vi "Create Write Channel.vi"(7 "Name":string, 8 "error in (no error)":errorcluster, 9 "Cluster":T1 {"Data Type" format="%.0x"}, 10 "Bitfile Name":string, 11 "Item Ref in":T3 format="%.0x") -> (0 "error out":errorcluster)   [LabVIEW 2018, in "FPGA Addon System Explorer.lvlib"]
uses:
  FPGA Addon System Explorer.lvlib
  <vilib>/NI Veristand/Custom Device API/Custom Device Item Ref.ctl
  Addon Shared/Types/Register Information.ctl
  Addon Shared/Types/Data Type.ctl
  <vilib>/NI Veristand/Custom Device API/Custom Device Channel.ctl
  <vilib>/NI Veristand/Custom Device API/Custom Device Channel Type.ctl
  Addon Shared/Types/FG Action.ctl
  niveristand-fpga-addon-speciality-io/Source/Types/PWM.Measure.Analog.Settings.ctl
  niveristand-fpga-addon-speciality-io/Source/Types/PWM.Generate.Digital.Convert.Settings.ctl
  niveristand-fpga-addon-speciality-io/Source/Types/PWM.Generate.Digital.Settings.ctl
  niveristand-fpga-addon-speciality-io/Source/Types/WSS.Generate.Digital.Convert.Settings.ctl
  niveristand-fpga-addon-speciality-io/Source/Types/WSS.Generate.Digital.Settings.ctl
  niveristand-fpga-addon-speciality-io/Source/Types/WSS.Sensor.Type.ctl
  niveristand-fpga-addon-speciality-io/Source/Types/Static.Generate.Digital.Settings.ctl
  niveristand-fpga-addon-speciality-io/Source/Types/Static.Measure.Digital.Settings.ctl
  niveristand-fpga-addon-speciality-io/Source/Types/Sine.Generate.Convert.Settings.ctl
  niveristand-fpga-addon-speciality-io/Source/Types/Sine.Generate.Settings.ctl
  niveristand-fpga-addon-speciality-io/Source/Types/PWM.Measure.Digital.Settings.ctl
  niveristand-fpga-addon-speciality-io/Source/Types/QuadratureEncoder.Measure.Digital.Settings.ctl
  niveristand-fpga-addon-speciality-io/Source/Types/QuadratureEncoder.Measure.Digital.Settings.Direction.ctl
  Addon Shared/SubVIs/Constants.vi
  <vilib>/NI/NI VeriStand Advanced SysDef API/SysDef API/SysDef.Property.Get.vi
  <vilib>/NI/NI VeriStand Advanced SysDef API/_SubVIs/SysDef.Property.Get.Variant.vi
  <vilib>/NI/NI VeriStand Advanced SysDef API/SysDef API/SysDef.Property.Set.vi
  <vilib>/NI/NI VeriStand Advanced SysDef API/_SubVIs/SysDef.Property.Set.Variant.vi
  <vilib>/NI Veristand/Custom Device API/Custom Device API.lvlib
  Addon Shared/FPGA Addon Shared.lvlib
  niveristand-fpga-addon-speciality-io/Source/Speciality FPGA IO.lvlib
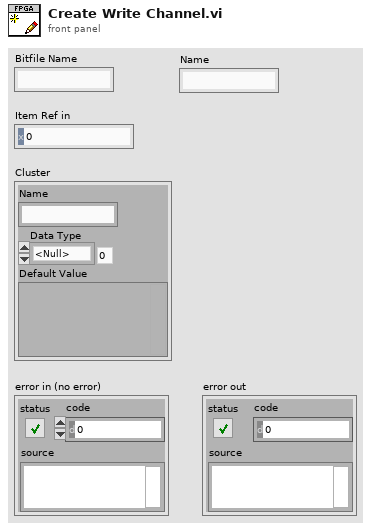
[diagram p1: front panel]
types:
  T1 = typedef "FPGA Addon Shared.lvlib/Register Information.ctl" = cluster{"Name":string, "Data Type":T2, "Default Value":variant}
  T2 = typedef "FPGA Addon Shared.lvlib/Data Type.ctl" = enum8{"<Null>", "I8", "I16", "I32", "I64", "U8", "U16", "U32", "U64", "SGL", "Boolean", "Analog PWM In Settings", "Analog PWM In", "Digital PWM In Settings", "Digital PWM In", "Digital PWM Out", "Sine Out", "FXP+/-24.5", "FXP+/-16.5", "FXP+/-32.8", "FXP+/-64.32", "FXP+/-16.7", "FXP+/-20.5", "FXP+/-27.5", "FXP+/-32.16", "FXP+16.3", "FXP+18.3", "Digital Static In", "Digital Static Out", "Digital Static In Settings", "Digital WSS Out", "Quad Encoder Settings", "Quad Encoder In", "Group"}
  T3 = typedef "Custom Device API.lvlib/Custom Device Item Ref.ctl" = u64
  T4 = typedef "Custom Device API.lvlib/Custom Device Channel.ctl" = cluster{"Type":T5, "Units":string, "Default Value":dbl, "Faultable":bool, "Scalable":bool}
  T5 = typedef "Custom Device API.lvlib/Custom Device Channel Type.ctl" = enum16{"Input", "Output"}
  T6 = typedef "FPGA Addon Shared.lvlib/FG Action.ctl" = enum8{"GET", "SET"}
  T7 = typedef "Speciality FPGA IO.lvlib/PWM.Measure.Analog.Settings.ctl" = cluster{"ACTIVE EDGE":bool, "TIMEOUT":u32, "THRESHOLD":fxp<+/-,32,8>}
  T8 = typedef "Speciality FPGA IO.lvlib/PWM.Generate.Digital.Convert.Settings.ctl" = cluster{"ACTIVE EDGE":bool, "FREQ":sgl, "DC":sgl}
  T9 = typedef "Speciality FPGA IO.lvlib/PWM.Generate.Digital.Settings.ctl" = cluster{"ACTIVE EDGE":bool, "ACTIVE TICKS":u32, "INACTIVE TICKS":u32}
  T10 = typedef "Speciality FPGA IO.lvlib/WSS.Generate.Digital.Convert.Settings.ctl" = cluster{"SPEED":u32, "DATA":u8, "PPR":u32, "WD":u32, "TYPE":u8}
  T11 = typedef "Speciality FPGA IO.lvlib/WSS.Generate.Digital.Settings.ctl" = cluster{"ACTIVE EDGE":bool, "ACTIVE TICKS":u32, "INACTIVE TICKS":u32, "DATA":u8, "SENSOR TYPE":u8}
  T12 = typedef "Speciality FPGA IO.lvlib/WSS.Sensor.Type.ctl" = enum16{"Unidirectional", "Bosch Bidirectional", "Continental Bidirectional"}
  T13 = typedef "Speciality FPGA IO.lvlib/Sine.Generate.Convert.Settings.ctl" = cluster{"AMP":sgl, "OFFSET":sgl, "FREQ":sgl}
  T14 = typedef "Speciality FPGA IO.lvlib/Sine.Generate.Settings.ctl" = cluster{"AMP":fxp<+/-,32,8>, "OFFSET":fxp<+/-,32,8>, "PERIODS/TICKS":fxp<+,32,0>}
  T15 = typedef "Speciality FPGA IO.lvlib/QuadratureEncoder.Measure.Digital.Settings.Direction.ctl" = enum16{"Increment A Leads B", "Increment B Leads A"}
  T16 = typedef "Speciality FPGA IO.lvlib/Static.Generate.Digital.Settings.ctl" = cluster{"ACTIVE EDGE":bool, "OUTPUT":bool}
  T17 = typedef "Speciality FPGA IO.lvlib/Static.Measure.Digital.Settings.ctl" = cluster{"ACTIVE EDGE":bool}
  T18 = typedef "Speciality FPGA IO.lvlib/PWM.Measure.Digital.Settings.ctl" = cluster{"ACTIVE EDGE":bool, "TIMEOUT":u32}
  T19 = typedef "Speciality FPGA IO.lvlib/QuadratureEncoder.Measure.Digital.Settings.ctl" = cluster{"DIRECTION":u8, "RESET VALUE":i32, "A RESET STATE":bool, "B RESET STATE":bool, "Z RESET STATE":bool}
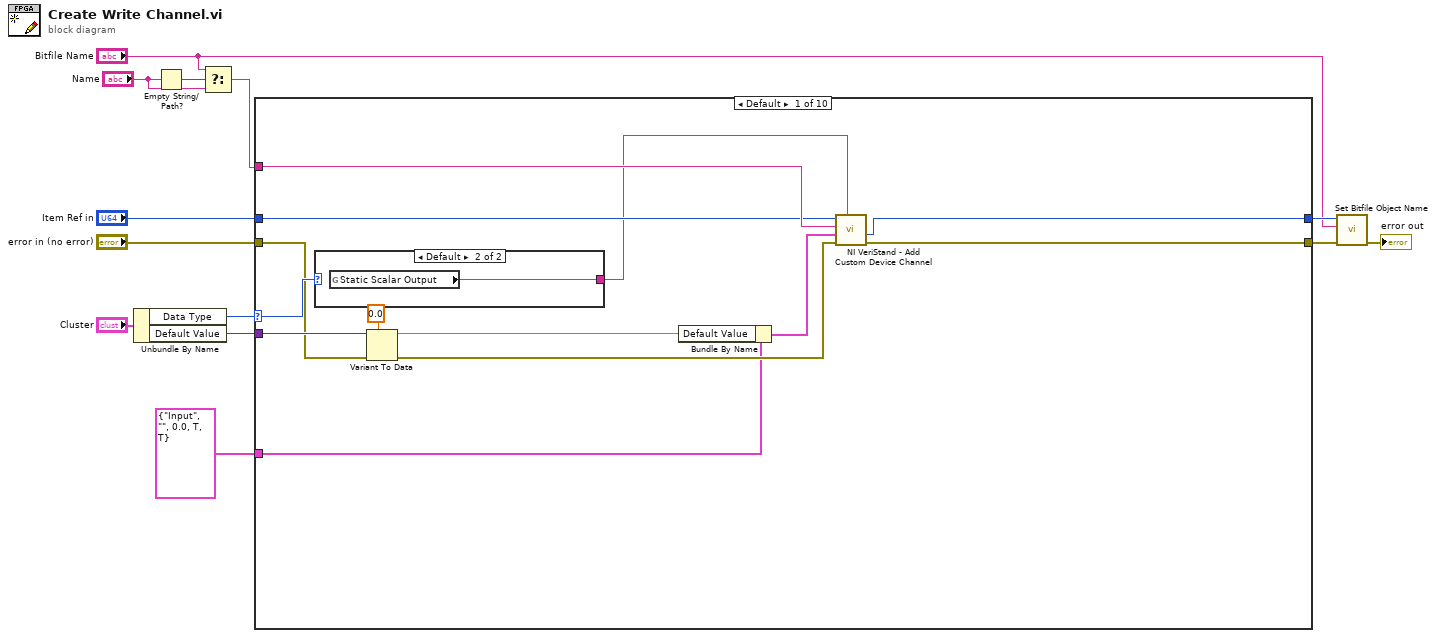
[diagram p0: block diagram]
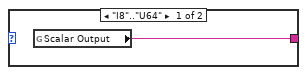
[diagram p2: hidden frame]
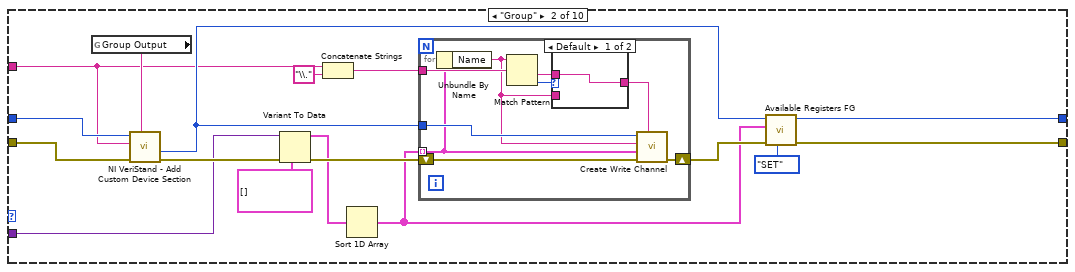
[diagram p3: hidden frame]
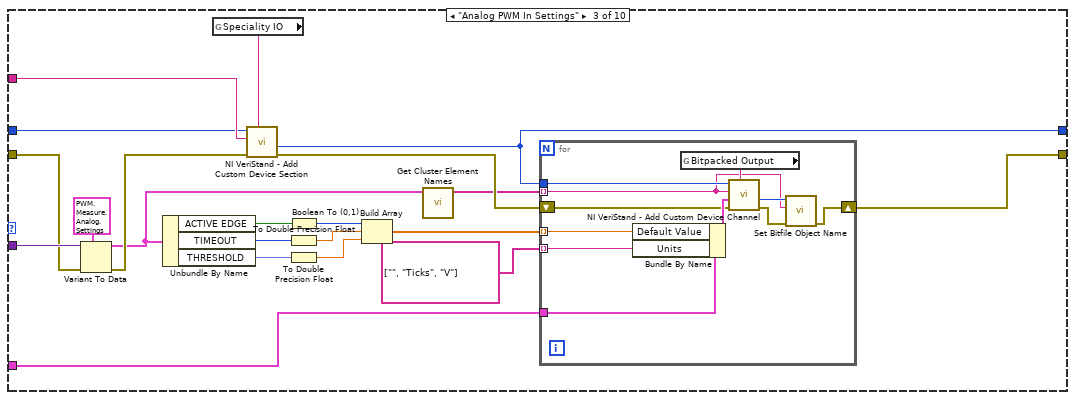
[diagram p5: hidden frame]
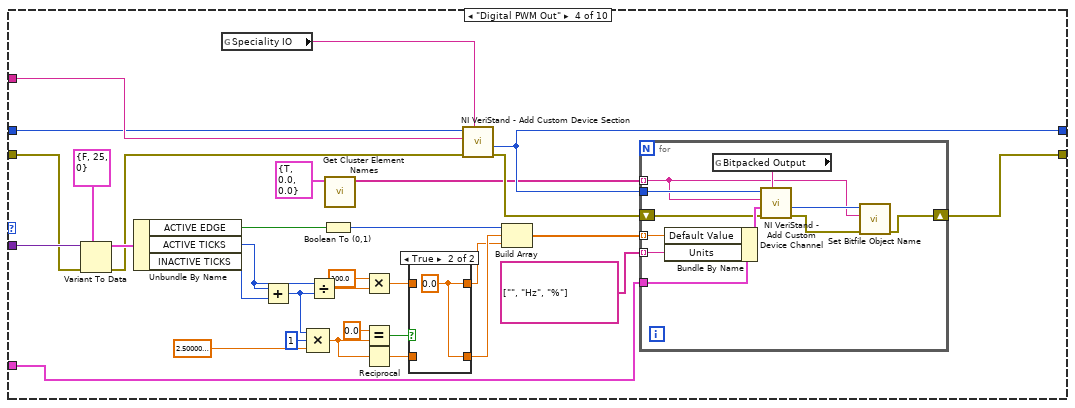
[diagram p6: hidden frame]
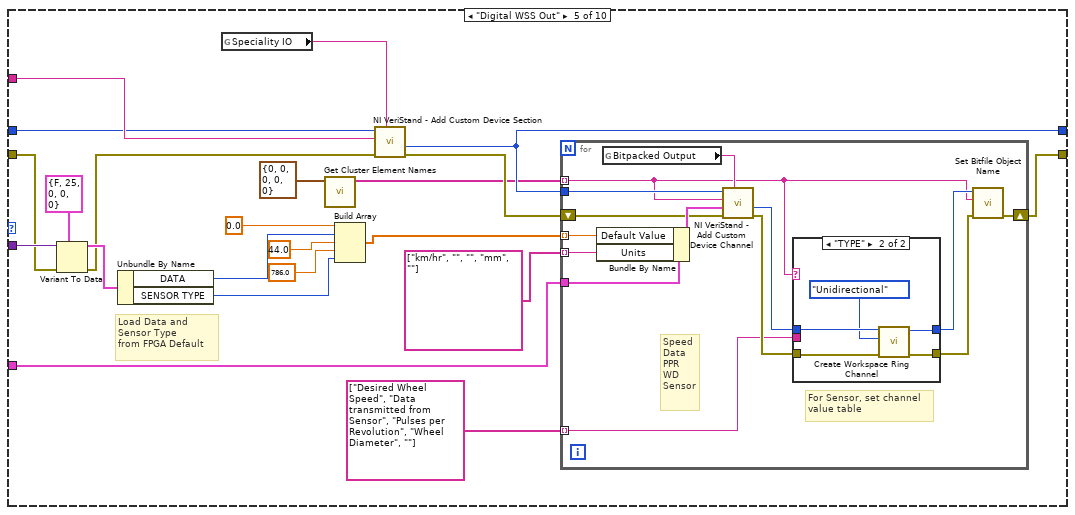
[diagram p8: hidden frame]
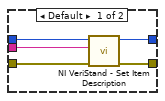
[diagram p9: hidden frame]
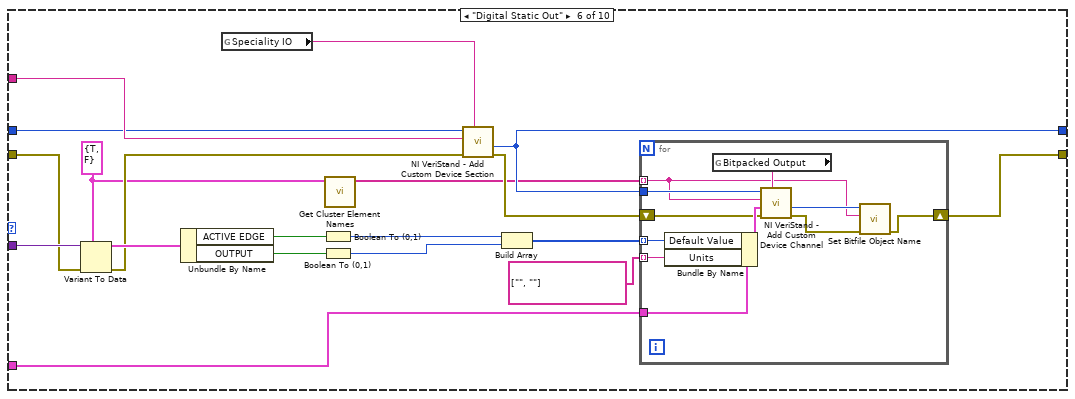
[diagram p10: hidden frame]
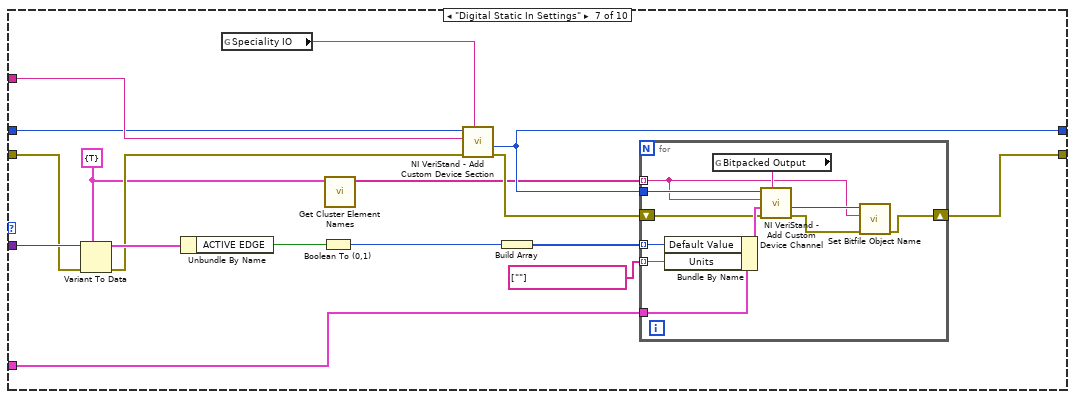
[diagram p11: hidden frame]
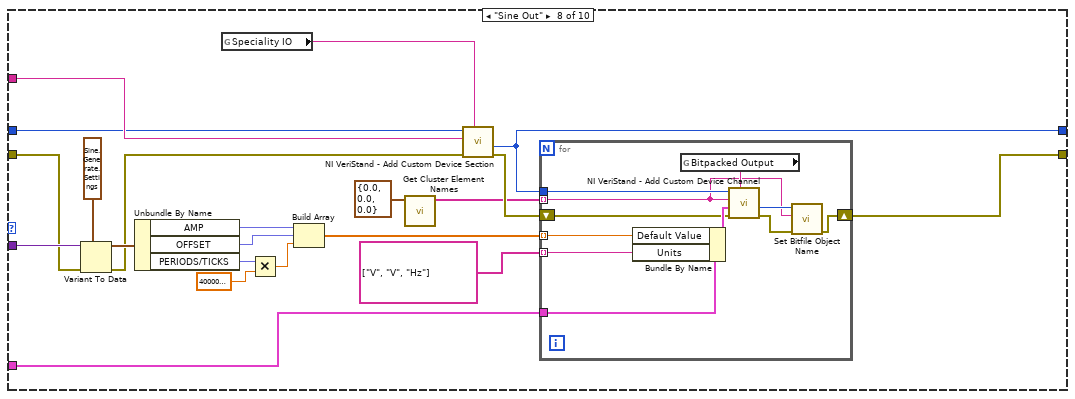
[diagram p12: hidden frame]
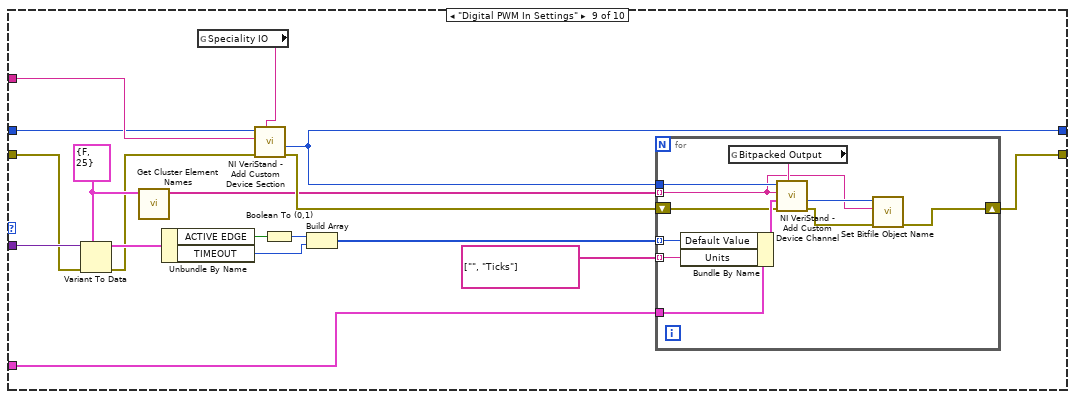
[diagram p13: hidden frame]
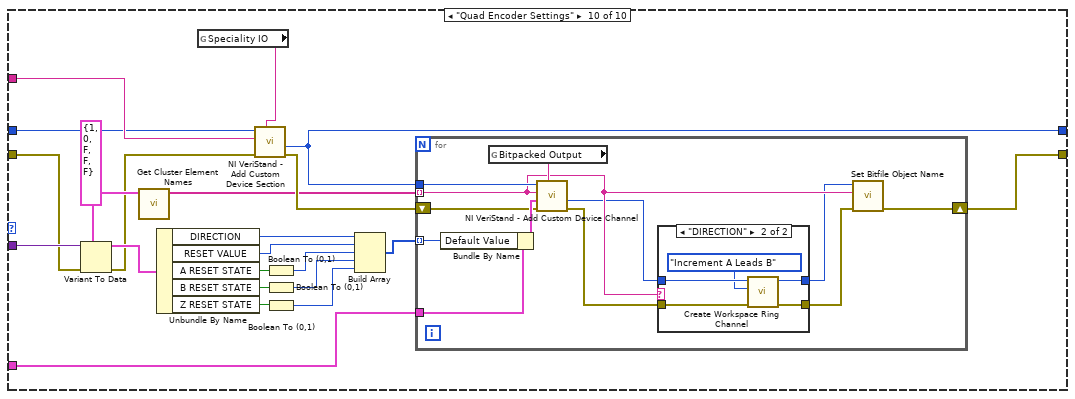
[diagram p14: hidden frame]
diagram:
  n1 = Unbundle By Name("Cluster") -> ("Data Type"=w9:T2, "Default Value"=w8:variant)
  n2 = Empty String/Path?(string/path="Name") -> (empty?=w4:bool)
  n3 = Select(t="Bitfile Name", s=w4, f="Name") -> (s? t:f=w1:string)
  n4 = case shown="Default" w9 {
    selector: w9 -> [w20 _ _ _ _ _ _ _ _ _]
    tunnel: [w26 w34 w71 w114 w150 w193 w221 w253 w282 w315] -> w12
    tunnel: w1 -> [w25 w30 w77 w120 w156 w199 w227 w259 w288 w321]
    tunnel: [w24 w36 w70 w116 w152 w195 w223 w255 w284 w317] -> w11
    tunnel: "Item Ref in" -> [w23 w40 w76 w119 w155 w198 w226 w258 w287 w320]
    tunnel: "error in (no error)" -> [w16 w41 w74 w117 w153 w196 w224 w256 w285 w318]
    tunnel: w8 -> [w19 w39 w75 w118 w154 w197 w225 w257 w286 w319]
    tunnel: T4 {"Type"=enum."Input", "Units"="", "Default Value"=0.0, "Faultable"=TRUE, "Scalable"=TRUE} ("Channel") -> [w14 _ w57 w89 w141 w181 w211 w239 w271 w307]
    frame Default {
      n5 = case shown="Default" w20 {
        tunnel: [w27 w28] -> w22
        frame "I8".."U64" {
          n6 = global read "Constants.vi" "Scalar Output"() -> (w27:string)
        }
        frame Default {
          n7 = global read "Constants.vi" "Static Scalar Output"() -> (w28:string)
        }
      }
      n8 = Variant To Data(error in=w16, type=0.0 ("Default Value"), Variant=w19) -> (data=w17:dbl, error out=w15:errorcluster)
      n9 = Bundle By Name(cluster=w14, "Default Value"=w17) -> (w21:T4)
      n10 = call <vilib>:"NI VeriStand - Add Custom Device Channel.vi"("GUID (Default Channel)"=w22, "error in (no error)"=w15, "Channel"=w21, "Channel Name"=w25, "Parent Ref in"=w23) -> ("error out"=w26:errorcluster, "Channel Ref"=w24:T3)  [unwired: 3 in, 2 out]
    }
    frame "Group" {
      n11 = global read "Constants.vi" "Group Output"() -> (w43:string)
      n12 = call <vilib>:"NI VeriStand - Add Custom Device Section.vi"("GUID (Default Section)"=w43, "error in (no error)"=w41, "Section Name"=w30, "Parent Ref in"=w40) -> ("error out"=w42:errorcluster, "Section Ptr"=w37:T3)  [unwired: 4 in, 2 out]
      n13 = Variant To Data(error in=w42, type=T1[] [], Variant=w39) -> (data=w33:T1[], error out=w44:errorcluster)
      n14 = Concatenate Strings(w30, "\\.") -> (w29:string)
      n15 = Sort 1D Array(array=w33) -> (sorted array=w32:T1[])
      n16 = for {
        tunnel: w32 -> [w48] mode=indexing
        shift-right: [w52] -> w35
        shift-left: w44 -> [w54]
        tunnel: w37 -> [w53]
        tunnel: w29 -> [w49]
        n17 = Unbundle By Name(w48) -> ("Name"=w47:string)
        n18 = Match Pattern(string=w47, regular expression=w49) -> (after substring=w50:string, offset past match=w51:i32)  [unwired: 1 in, 2 out]
        n19 = case shown="Default" w51 {
          tunnel: [w55 w56] -> w46
          tunnel: w50 -> [w55 _]
          tunnel: w47 -> [_ w56]
          frame Default {
          }
          frame -1 {
          }
        }
        n20 = call "Create Write Channel.vi"("Name"=w46, "error in (no error)"=w54, "Cluster"=w48, "Bitfile Name"=w47, "Item Ref in"=w53) -> ("error out"=w52:errorcluster)  [unwired: 6 in]
      }
      n21 = call "Available Registers FG.vi"("Action"=FG_Action."SET", "error in (no error)"=w35, "Available Registers"=w32, "Item Ref"=w37) -> ("error out"=w34:errorcluster, "Item Ref out"=w36:T3)  [unwired: 5 in, 1 out]
    }
    frame "Analog PWM In Settings" {
      n22 = Variant To Data(error in=w74, type=T7 {"ACTIVE EDGE"=FALSE, "TIMEOUT"=1000000000, "THRESHOLD"=25.0} ("Channel.Settings"), Variant=w75) -> (data=w59:T7, error out=w60:errorcluster)
      n23 = Unbundle By Name(w59) -> ("ACTIVE EDGE"=w65:bool, "TIMEOUT"=w69:u32, "THRESHOLD"=w64:fxp<+/-,32,8>)
      n24 = global read "Constants.vi" "Speciality IO"() -> (w61:string)
      n25 = call <vilib>:"NI VeriStand - Add Custom Device Section.vi"("GUID (Default Section)"=w61, "error in (no error)"=w60, "Section Name"=w77, "Parent Ref in"=w76) -> ("error out"=w72:errorcluster, "Section Ptr"=w70:T3)  [unwired: 4 in, 2 out]
      n26 = Boolean To (0,1)(Boolean=w65) -> (0, 1=w63:i16)
      n27 = To Double Precision Float(number=w69) -> (double precision float=w67:dbl)
      n28 = To Double Precision Float(number=w64) -> (double precision float=w62:dbl)
      n29 = Build Array(w63, w67, w62) -> (w68:dbl[])
      n30 = call "Get Cluster Element Names.vi"("Cluster"=w59) -> ("Channels"=w58:string[])  [unwired: 10 in]
      n31 = for {
        tunnel: w70 -> [w87]
        shift-right: [w80] -> w71
        shift-left: w72 -> [w86]
        tunnel: w68 -> [w84] mode=indexing
        tunnel: string[] ["", "Ticks", "V"] -> [w83] mode=indexing
        tunnel: w58 -> [w79] mode=indexing
        tunnel: w57 -> [w78]
        n32 = Bundle By Name(cluster=w78, "Default Value"=w84, "Units"=w83) -> (w88:T4)
        n33 = global read "Constants.vi" "Bitpacked Output"() -> (w85:string)
        n34 = call <vilib>:"NI VeriStand - Add Custom Device Channel.vi"("GUID (Default Channel)"=w85, "error in (no error)"=w86, "Channel"=w88, "Channel Name"=w79, "Parent Ref in"=w87) -> ("error out"=w81:errorcluster, "Channel Ref"=w82:T3)  [unwired: 3 in, 2 out]
        n35 = call "Set Bitfile Object Name.vi"("error in (no error)"=w81, "Name"=w79, "Channel Ref"=w82) -> ("error out"=w80:errorcluster)  [unwired: 8 in]
      }
    }
    frame "Digital PWM Out" {
      n36 = Variant To Data(error in=w117, type=T9 {"ACTIVE EDGE"=FALSE, "ACTIVE TICKS"=25, "INACTIVE TICKS"=0} ("Channel.Settings"), Variant=w118) -> (data=w113:T9, error out=w106:errorcluster)
      n37 = Unbundle By Name(w113) -> ("ACTIVE EDGE"=w112:bool, "ACTIVE TICKS"=w97:u32, "INACTIVE TICKS"=w96:u32)
      n38 = global read "Constants.vi" "Speciality IO"() -> (w109:string)
      n39 = Add(x=w97, y=w96) -> (x+y=w103:u32)
      n40 = Compound Arithmetic op=MULTIPLY(w103, u32 1 ("value"), 2.5000000292152436e-08 ("y")) -> (w104:dbl)
      n41 = Divide(x=w97, y=w103) -> (x/y=w99:dbl)
      n42 = Boolean To (0,1)(Boolean=w112) -> (0, 1=w111:i16)
      n43 = call "Get Cluster Element Names.vi"("Cluster"=T8 {"ACTIVE EDGE"=TRUE, "FREQ"=0.0, "DC"=0.0} ("Settings")) -> ("Channels"=w107:string[])  [unwired: 10 in]
      n44 = Multiply(x=100.0, y=w99) -> (x*y=w91:dbl)
      n45 = Equal?(x=0.0, y=w104) -> (x = y?=w95:bool)
      n46 = Reciprocal(x=w104) -> (1/x=w93:dbl)
      n47 = case shown="True" w95 {
        tunnel: [w122 w123] -> w94
        tunnel: w93 -> [w122 _]
        tunnel: [w121 w123] -> w92
        tunnel: w91 -> [w121 _]
        frame False {
        }
        frame True {
          w123 = 0.0
        }
      }
      n48 = call <vilib>:"NI VeriStand - Add Custom Device Section.vi"("GUID (Default Section)"=w109, "error in (no error)"=w106, "Section Name"=w120, "Parent Ref in"=w119) -> ("error out"=w115:errorcluster, "Section Ptr"=w116:T3)  [unwired: 4 in, 2 out]
      n49 = Build Array(w111, w94, w92) -> (w110:dbl[])
      n50 = for {
        tunnel: w116 -> [w133]
        shift-right: [w126] -> w114
        shift-left: w115 -> [w132]
        tunnel: w110 -> [w130] mode=indexing
        tunnel: w107 -> [w125] mode=indexing
        tunnel: string[] ["", "Hz", "%"] -> [w129] mode=indexing
        tunnel: w89 -> [w124]
        n51 = Bundle By Name(cluster=w124, "Default Value"=w130, "Units"=w129) -> (w134:T4)
        n52 = global read "Constants.vi" "Bitpacked Output"() -> (w131:string)
        n53 = call <vilib>:"NI VeriStand - Add Custom Device Channel.vi"("GUID (Default Channel)"=w131, "error in (no error)"=w132, "Channel"=w134, "Channel Name"=w125, "Parent Ref in"=w133) -> ("error out"=w127:errorcluster, "Channel Ref"=w128:T3)  [unwired: 3 in, 2 out]
        n54 = call "Set Bitfile Object Name.vi"("error in (no error)"=w127, "Name"=w125, "Channel Ref"=w128) -> ("error out"=w126:errorcluster)  [unwired: 8 in]
      }
    }
    frame "Digital WSS Out" {
      # "Load Data and\nSensor Type\nfrom FPGA Default"
      n55 = Variant To Data(error in=w153, type=T11 {"ACTIVE EDGE"=FALSE, "ACTIVE TICKS"=25, "INACTIVE TICKS"=0, "DATA"=0, "SENSOR TYPE"=0} ("Channel.Settings"), Variant=w154) -> (data=w149:T11, error out=w144:errorcluster)
      n56 = Unbundle By Name(w149) -> ("DATA"=w135:u8, "SENSOR TYPE"=w136:u8)
      n57 = global read "Constants.vi" "Speciality IO"() -> (w147:string)
      n58 = call "Get Cluster Element Names.vi"("Cluster"=T10 {"SPEED"=0, "DATA"=0, "PPR"=0, "WD"=0, "TYPE"=0} ("Wheel Speed Sensor Settings")) -> ("Channels"=w145:string[])  [unwired: 10 in]
      n59 = Build Array(0.0 ("element"), w135, 44.0 ("element"), 786.0 ("element"), w136) -> (w148:dbl[])
      n60 = call <vilib>:"NI VeriStand - Add Custom Device Section.vi"("GUID (Default Section)"=w147, "error in (no error)"=w144, "Section Name"=w156, "Parent Ref in"=w155) -> ("error out"=w151:errorcluster, "Section Ptr"=w152:T3)  [unwired: 4 in, 2 out]
      n61 = for {
        tunnel: w152 -> [w169]
        shift-right: [w164] -> w150
        shift-left: w151 -> [w168]
        tunnel: w148 -> [w166] mode=indexing
        tunnel: w145 -> [w157] mode=indexing
        tunnel: string[] ["km/hr", "", "", "mm", ""] -> [w165] mode=indexing
        tunnel: w141 -> [w163]
        tunnel: string[] ["Desired Wheel Speed", "Data transmitted from Sensor", "Pulses per Revolution", "Wheel Diameter", ""] -> [w158] mode=indexing
        # "For Sensor, set channel \nvalue table"
        # "Speed\nData\nPPR\nWD\nSensor"
        n62 = Bundle By Name(cluster=w163, "Default Value"=w166, "Units"=w165) -> (w170:T4)
        n63 = global read "Constants.vi" "Bitpacked Output"() -> (w167:string)
        n64 = call <vilib>:"NI VeriStand - Add Custom Device Channel.vi"("GUID (Default Channel)"=w167, "error in (no error)"=w168, "Channel"=w170, "Channel Name"=w157, "Parent Ref in"=w169) -> ("error out"=w162:errorcluster, "Channel Ref"=w160:T3)  [unwired: 3 in, 2 out]
        n65 = case shown="\"TYPE\"" w157 {
          tunnel: w162 -> [w175 w179]
          tunnel: [w174 w178] -> w161
          tunnel: w160 -> [w173 w180]
          tunnel: [w172 w177] -> w159
          tunnel: w158 -> [w171 _]
          frame Default {
            n66 = call <vilib>:"NI VeriStand - Set Item Description.vi"("error in (no error)"=w175, "Description"=w171, "Item Ref in"=w173) -> ("error out"=w174:errorcluster, "Item Ref out"=w172:T3)  [unwired: 6 in, 1 out]
          }
          frame "TYPE" {
            n67 = call "Create Workspace Ring Channel.vi"("error in (no error)"=w179, "Enum"=WSS.Sensor.Type."Unidirectional" ("Sensor Type"), "Channel Ref in"=w180) -> ("error out"=w178:errorcluster, "Channel Ref out"=w177:T3)  [unwired: 7 in]
          }
        }
        n68 = call "Set Bitfile Object Name.vi"("error in (no error)"=w161, "Name"=w157, "Channel Ref"=w159) -> ("error out"=w164:errorcluster)  [unwired: 8 in]
      }
    }
    frame "Digital Static Out" {
      w184 = T16 {"ACTIVE EDGE"=TRUE, "OUTPUT"=FALSE} ("Settings")
      n69 = Variant To Data(error in=w196, type=w184, Variant=w197) -> (data=w192:T16, error out=w186:errorcluster)
      n70 = Unbundle By Name(w192) -> ("ACTIVE EDGE"=w191:bool, "OUTPUT"=w183:bool)
      n71 = global read "Constants.vi" "Speciality IO"() -> (w188:string)
      n72 = Boolean To (0,1)(Boolean=w191) -> (0, 1=w190:i16)
      n73 = Boolean To (0,1)(Boolean=w183) -> (0, 1=w182:i16)
      n74 = call "Get Cluster Element Names.vi"("Cluster"=w184) -> ("Channels"=w187:string[])  [unwired: 10 in]
      n75 = call <vilib>:"NI VeriStand - Add Custom Device Section.vi"("GUID (Default Section)"=w188, "error in (no error)"=w186, "Section Name"=w199, "Parent Ref in"=w198) -> ("error out"=w194:errorcluster, "Section Ptr"=w195:T3)  [unwired: 4 in, 2 out]
      n76 = Build Array(w190, w182) -> (w189:i16[])
      n77 = for {
        tunnel: w195 -> [w209]
        shift-right: [w202] -> w193
        shift-left: w194 -> [w208]
        tunnel: w189 -> [w206] mode=indexing
        tunnel: w187 -> [w201] mode=indexing
        tunnel: string[] ["", ""] -> [w205] mode=indexing
        tunnel: w181 -> [w200]
        n78 = Bundle By Name(cluster=w200, "Default Value"=w206, "Units"=w205) -> (w210:T4)
        n79 = global read "Constants.vi" "Bitpacked Output"() -> (w207:string)
        n80 = call <vilib>:"NI VeriStand - Add Custom Device Channel.vi"("GUID (Default Channel)"=w207, "error in (no error)"=w208, "Channel"=w210, "Channel Name"=w201, "Parent Ref in"=w209) -> ("error out"=w203:errorcluster, "Channel Ref"=w204:T3)  [unwired: 3 in, 2 out]
        n81 = call "Set Bitfile Object Name.vi"("error in (no error)"=w203, "Name"=w201, "Channel Ref"=w204) -> ("error out"=w202:errorcluster)  [unwired: 8 in]
      }
    }
    frame "Digital Static In Settings" {
      w212 = T17 {"ACTIVE EDGE"=TRUE} ("Settings")
      n82 = Variant To Data(error in=w224, type=w212, Variant=w225) -> (data=w220:T17, error out=w214:errorcluster)
      n83 = Unbundle By Name(w220) -> ("ACTIVE EDGE"=w219:bool)
      n84 = global read "Constants.vi" "Speciality IO"() -> (w216:string)
      n85 = Boolean To (0,1)(Boolean=w219) -> (0, 1=w218:i16)
      n86 = call "Get Cluster Element Names.vi"("Cluster"=w212) -> ("Channels"=w215:string[])  [unwired: 10 in]
      n87 = call <vilib>:"NI VeriStand - Add Custom Device Section.vi"("GUID (Default Section)"=w216, "error in (no error)"=w214, "Section Name"=w227, "Parent Ref in"=w226) -> ("error out"=w222:errorcluster, "Section Ptr"=w223:T3)  [unwired: 4 in, 2 out]
      n88 = Build Array(w218) -> (w217:i16[])
      n89 = for {
        tunnel: w223 -> [w237]
        shift-right: [w230] -> w221
        shift-left: w222 -> [w236]
        tunnel: w217 -> [w234] mode=indexing
        tunnel: w215 -> [w229] mode=indexing
        tunnel: string[] [""] -> [w233] mode=indexing
        tunnel: w211 -> [w228]
        n90 = Bundle By Name(cluster=w228, "Default Value"=w234, "Units"=w233) -> (w238:T4)
        n91 = global read "Constants.vi" "Bitpacked Output"() -> (w235:string)
        n92 = call <vilib>:"NI VeriStand - Add Custom Device Channel.vi"("GUID (Default Channel)"=w235, "error in (no error)"=w236, "Channel"=w238, "Channel Name"=w229, "Parent Ref in"=w237) -> ("error out"=w231:errorcluster, "Channel Ref"=w232:T3)  [unwired: 3 in, 2 out]
        n93 = call "Set Bitfile Object Name.vi"("error in (no error)"=w231, "Name"=w229, "Channel Ref"=w232) -> ("error out"=w230:errorcluster)  [unwired: 8 in]
      }
    }
    frame "Sine Out" {
      n94 = Variant To Data(error in=w256, type=T14 {"AMP"=0.0, "OFFSET"=0.0, "PERIODS/TICKS"=0.0} ("Settings"), Variant=w257) -> (data=w252:T14, error out=w247:errorcluster)
      n95 = Unbundle By Name(w252) -> ("AMP"=w245:fxp<+/-,32,8>, "OFFSET"=w244:fxp<+/-,32,8>, "PERIODS/TICKS"=w243:fxp<+,32,0>)
      n96 = global read "Constants.vi" "Speciality IO"() -> (w250:string)
      n97 = Multiply(x=w243, y=sgl 40000000.0) -> (x*y=w241:sgl)
      n98 = Build Array(w245, w244, w241) -> (w251:sgl[])
      n99 = call "Get Cluster Element Names.vi"("Cluster"=T13 {"AMP"=0.0, "OFFSET"=0.0, "FREQ"=0.0} ("Settings")) -> ("Channels"=w248:string[])  [unwired: 10 in]
      n100 = call <vilib>:"NI VeriStand - Add Custom Device Section.vi"("GUID (Default Section)"=w250, "error in (no error)"=w247, "Section Name"=w259, "Parent Ref in"=w258) -> ("error out"=w254:errorcluster, "Section Ptr"=w255:T3)  [unwired: 4 in, 2 out]
      n101 = for {
        tunnel: w255 -> [w269]
        shift-right: [w262] -> w253
        shift-left: w254 -> [w268]
        tunnel: w251 -> [w266] mode=indexing
        tunnel: w248 -> [w261] mode=indexing
        tunnel: string[] ["V", "V", "Hz"] -> [w265] mode=indexing
        tunnel: w239 -> [w260]
        n102 = Bundle By Name(cluster=w260, "Default Value"=w266, "Units"=w265) -> (w270:T4)
        n103 = global read "Constants.vi" "Bitpacked Output"() -> (w267:string)
        n104 = call <vilib>:"NI VeriStand - Add Custom Device Channel.vi"("GUID (Default Channel)"=w267, "error in (no error)"=w268, "Channel"=w270, "Channel Name"=w261, "Parent Ref in"=w269) -> ("error out"=w263:errorcluster, "Channel Ref"=w264:T3)  [unwired: 3 in, 2 out]
        n105 = call "Set Bitfile Object Name.vi"("error in (no error)"=w263, "Name"=w261, "Channel Ref"=w264) -> ("error out"=w262:errorcluster)  [unwired: 8 in]
      }
    }
    frame "Digital PWM In Settings" {
      w275 = T18 {"ACTIVE EDGE"=FALSE, "TIMEOUT"=25} ("Channel.Settings")
      n106 = Variant To Data(error in=w285, type=w275, Variant=w286) -> (data=w278:T18, error out=w273:errorcluster)
      n107 = call "Get Cluster Element Names.vi"("Cluster"=w275) -> ("Channels"=w274:string[])  [unwired: 10 in]
      n108 = Unbundle By Name(w278) -> ("ACTIVE EDGE"=w281:bool, "TIMEOUT"=w280:u32)
      n109 = global read "Constants.vi" "Speciality IO"() -> (w276:string)
      n110 = call <vilib>:"NI VeriStand - Add Custom Device Section.vi"("GUID (Default Section)"=w276, "error in (no error)"=w273, "Section Name"=w288, "Parent Ref in"=w287) -> ("error out"=w283:errorcluster, "Section Ptr"=w284:T3)  [unwired: 4 in, 2 out]
      n111 = Boolean To (0,1)(Boolean=w281) -> (0, 1=w279:i16)
      n112 = Build Array(w279, w280) -> (w277:u32[])
      n113 = for {
        tunnel: w284 -> [w298]
        shift-right: [w292] -> w282
        shift-left: w283 -> [w297]
        tunnel: w277 -> [w295] mode=indexing
        tunnel: w274 -> [w290] mode=indexing
        tunnel: string[] ["", "Ticks"] -> [w294] mode=indexing
        tunnel: w271 -> [w289]
        n114 = Bundle By Name(cluster=w289, "Default Value"=w295, "Units"=w294) -> (w299:T4)
        n115 = global read "Constants.vi" "Bitpacked Output"() -> (w296:string)
        n116 = call <vilib>:"NI VeriStand - Add Custom Device Channel.vi"("GUID (Default Channel)"=w296, "error in (no error)"=w297, "Channel"=w299, "Channel Name"=w290, "Parent Ref in"=w298) -> ("error out"=w293:errorcluster, "Channel Ref"=w291:T3)  [unwired: 3 in, 2 out]
        n117 = call "Set Bitfile Object Name.vi"("error in (no error)"=w293, "Name"=w290, "Channel Ref"=w291) -> ("error out"=w292:errorcluster)  [unwired: 8 in]
      }
    }
    frame "Quad Encoder Settings" {
      w310 = T19 {"DIRECTION"=1, "RESET VALUE"=0, "A RESET STATE"=FALSE, "B RESET STATE"=FALSE, "Z RESET STATE"=FALSE} ("Channel.Settings")
      n118 = Variant To Data(error in=w318, type=w310, Variant=w319) -> (data=w313:T19, error out=w308:errorcluster)
      n119 = call "Get Cluster Element Names.vi"("Cluster"=w310) -> ("Channels"=w309:string[])  [unwired: 10 in]
      n120 = Unbundle By Name(w313) -> ("DIRECTION"=w306:u8, "RESET VALUE"=w314:i32, "A RESET STATE"=w305:bool, "B RESET STATE"=w303:bool, "Z RESET STATE"=w301:bool)
      n121 = global read "Constants.vi" "Speciality IO"() -> (w311:string)
      n122 = call <vilib>:"NI VeriStand - Add Custom Device Section.vi"("GUID (Default Section)"=w311, "error in (no error)"=w308, "Section Name"=w321, "Parent Ref in"=w320) -> ("error out"=w316:errorcluster, "Section Ptr"=w317:T3)  [unwired: 4 in, 2 out]
      n123 = Boolean To (0,1)(Boolean=w305) -> (0, 1=w304:i16)
      n124 = Boolean To (0,1)(Boolean=w303) -> (0, 1=w302:i16)
      n125 = Boolean To (0,1)(Boolean=w301) -> (0, 1=w300:i16)
      n126 = Build Array(w306, w314, w304, w302, w300) -> (w312:i32[])
      n127 = for {
        tunnel: w317 -> [w332]
        shift-right: [w322] -> w315
        shift-left: w316 -> [w331]
        tunnel: w312 -> [w329] mode=indexing
        tunnel: w309 -> [w327] mode=indexing
        tunnel: w307 -> [w328]
        n128 = Bundle By Name(cluster=w328, "Default Value"=w329) -> (w333:T4)
        n129 = global read "Constants.vi" "Bitpacked Output"() -> (w330:string)
        n130 = call <vilib>:"NI VeriStand - Add Custom Device Channel.vi"("GUID (Default Channel)"=w330, "error in (no error)"=w331, "Channel"=w333, "Channel Name"=w327, "Parent Ref in"=w332) -> ("error out"=w324:errorcluster, "Channel Ref"=w326:T3)  [unwired: 3 in, 2 out]
        n131 = case shown="\"DIRECTION\"" w327 {
          tunnel: [w334 w339] -> w323
          tunnel: w326 -> [w335 w340]
          tunnel: [w335 w338] -> w325
          tunnel: w324 -> [w334 w337]
          frame Default {
          }
          frame "DIRECTION" {
            n132 = call "Create Workspace Ring Channel.vi"("error in (no error)"=w337, "Enum"=QuadratureEncoder.Measure.Digital.Settings.Direction."Increment A Leads B", "Channel Ref in"=w340) -> ("error out"=w339:errorcluster, "Channel Ref out"=w338:T3)  [unwired: 7 in]
          }
        }
        n133 = call "Set Bitfile Object Name.vi"("error in (no error)"=w323, "Name"=w327, "Channel Ref"=w325) -> ("error out"=w322:errorcluster)  [unwired: 8 in]
      }
    }
  }
  n134 = call "Set Bitfile Object Name.vi"("error in (no error)"=w12, "Name"="Bitfile Name", "Channel Ref"=w11) -> ("error out"=→"error out":errorcluster)  [unwired: 8 in]
